vi "Event Last Ack.vi"(10 "Event Actor":refnum<class "Event Actor.lvclass">) -> (3 "Event Last Ack Msg out":refnum<class "Event Last Ack Msg.lvclass">)   [LabVIEW 2021, in "Event Last Ack.lvlib" / "Event Last Ack Msg.lvclass"]
uses:
  Event Last Ack Msg.lvclass
  Event Actor/Event Actor.lvclass
  Event Last Ack Msg.lvclass/Event Last Ack Msg.ctl
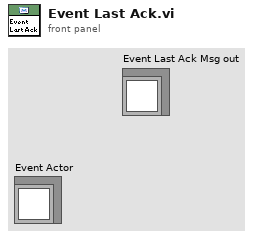
[diagram p1: front panel]
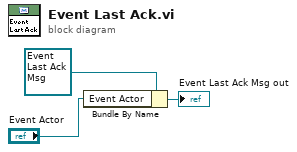
[diagram p0: block diagram]
diagram:
  n1 = Bundle By Name(cluster=refnum<class "Event Last Ack Msg.lvclass"> refnum ("Event Last Ack Msg out"), "Event Actor"="Event Actor") -> (→"Event Last Ack Msg out":refnum<class "Event Last Ack Msg.lvclass">)
